vi "SMU_gate_2_constant.vi"() -> ()   [LabVIEW 2022 SP3]
uses:
  <vilib>/Analysis/1siggen.llb/Ramp Pattern by Delta.vi
  Agilent U2722/Public/Configure/Configure Channel (Current).vi
  Agilent U2722/Public/Configure/Configure Channel (Voltage).vi
  Agilent U2722/Public/Data/Read Output (Single).vi
  <vilib>/Utility/file.llb/Write Delimited Spreadsheet (DBL).vi
  Agilent U2722/Agilent U2722.lvlib
  <vilib>/Analysis/NI_AALBase.lvlib
panel:
  in  "Tab Control":enum32{"Device Setup"}(tab)
  out "V_out (V)":dbl
  out "I_measure_channel (A)":dbl
  out "Vdd (V)":dbl
  in  "Voltage Range 2":u16(ring) items=["2 Volts", "20 Volts"]
  in  "Current Range 2":u16(ring)=4 items=["1 uA", "10 uA", "100 uA", "1 mA", "10 mA", "120 mA"]
  in  "Current Limit  2":dbl=0.005 format="%#_2p"
  in  "Voltage Range":u16(ring) items=["2 Volts", "20 Volts"]
  in  "Starting Voltage (V)":dbl
  in  "Stopping Voltage (V)":dbl=1.0
  in  "Voltage Interval  (DV)":dbl format="%#_2g"
  in  "Current Range":u16(ring)=4 items=["1 uA", "10 uA", "100 uA", "1 mA", "10 mA", "120 mA"]
  in  "VISA resource name SMU 1":refnum<visa-resource-name>
  in  "Gate 1 Channel Config":u16(ring)=1 items=["Channel 1"=1, "Channel 2"=2, "Channel 3"=3]
  in  "PLC":i32
  in  "Current Limit":dbl=0.005 format="%#_2p"
  in  "Interval Time (s)":dbl=1.0 caption="Delay Time (s)"
  in  "Vdd Channel Config":u16(ring)=2 items=["Channel 1"=1, "Channel 2"=2, "Channel 3"=3]
  in  "output file path":path
  out "XY Graph":cluster{"Y":dbl[], "Y":dbl[]}[](graph)
  in  "VISA resource name SMU 2":refnum<visa-resource-name>
  in  "Voltage Range 3":u16(ring) items=["2 Volts", "20 Volts"]
  in  "Current Range 3":u16(ring)=4 items=["1 uA", "10 uA", "100 uA", "1 mA", "10 mA", "120 mA"]
  in  "Gate 2 Channel Config":u16(ring)=1 items=["Channel 1"=1, "Channel 2"=2, "Channel 3"=3]
  in  "PLC 2":i32
  in  "Current Limit  3":dbl=0.005 format="%#_2p"
  in  "Output Measure Channel Config":u16(ring)=2 items=["Channel 1"=1, "Channel 2"=2, "Channel 3"=3]
  in  "Vdd (V)":dbl
  in  "Gate 2 Voltage (V)":dbl
  out "Idd (A)":dbl
  # "Gate 1 Sweep Settings"
  # "Vdd Voltage Setting"
  # "Should be 0!"
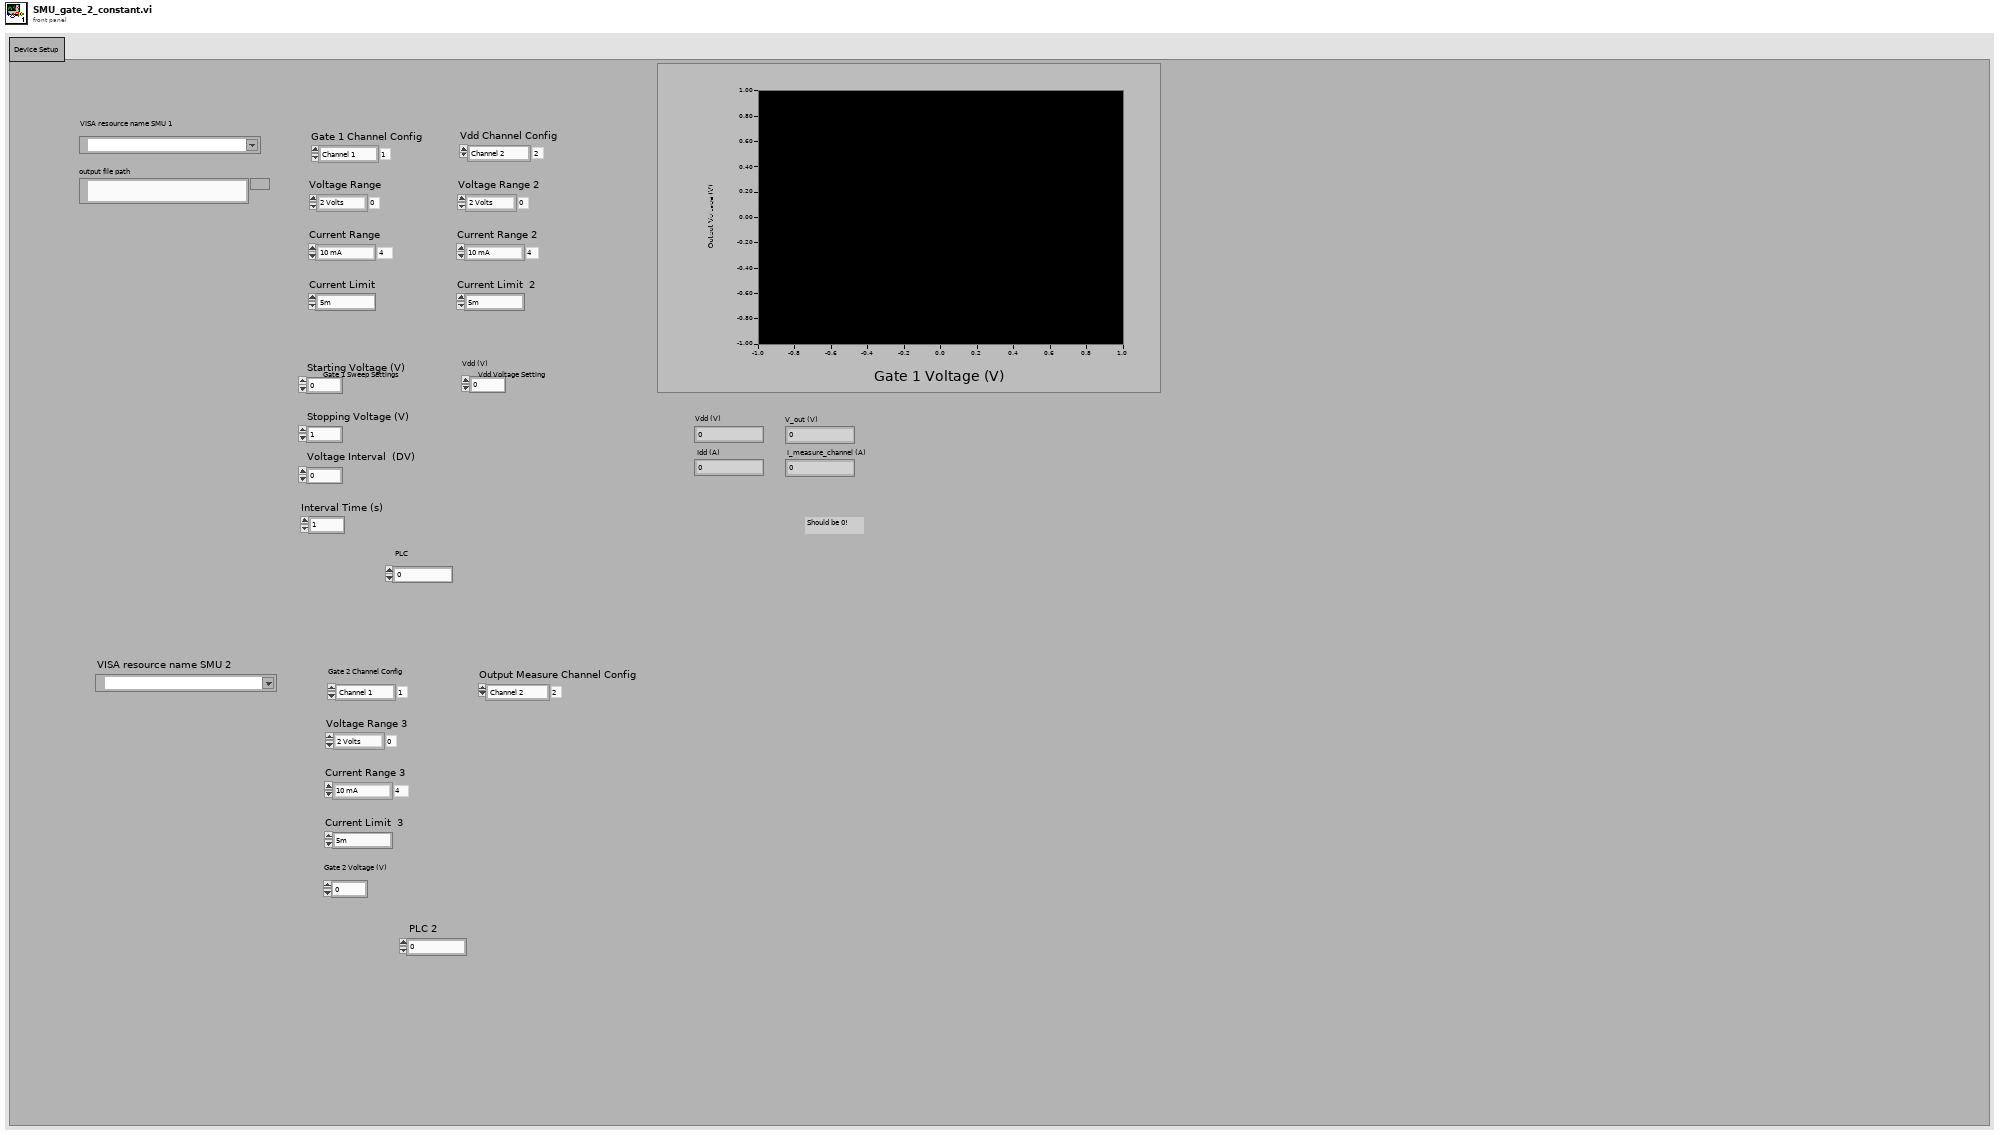
[diagram p1: front panel]
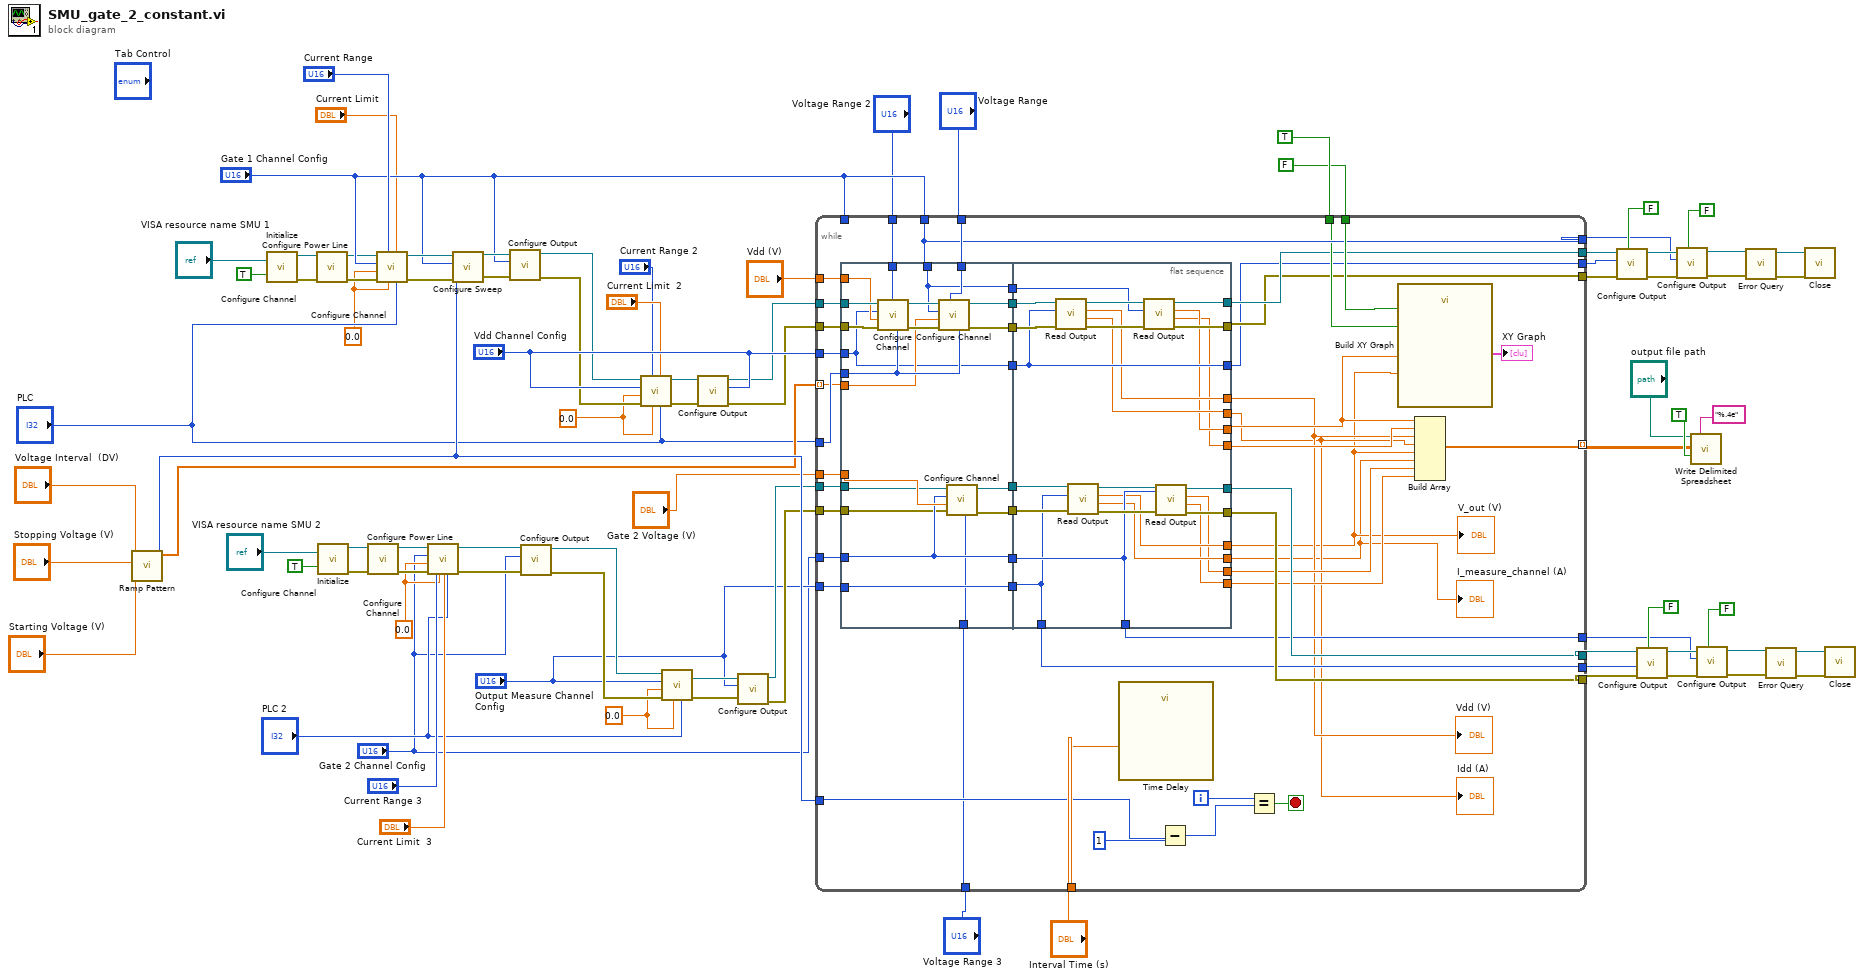
[diagram p0: block diagram]
diagram:
  w31 = 0.0
  w30 = 0.0
  w45 = 0.0
  w44 = 0.0
  n1 = call-poly <vilib>:"Ramp Pattern.vi"("start"="Starting Voltage (V)", "end"="Stopping Voltage (V)", "delta"="Voltage Interval  (DV)") -> ("samples"=w72:i32, "Ramp Pattern"=w64:dbl[])  [unwired: 6 in, 1 out]
  n2 = call "Initialize.vi"("ID Query (True)"=TRUE, "VISA resource name"="VISA resource name SMU 1") -> ("error out"=w82:errorcluster, "VISA resource name out"=w81:refnum<visa-resource-name>)  [unwired: 8 in]
  n3 = call "Configure Power Line.vi"("error in (no error)"=w82, "VISA resource name"=w81) -> ("error out"=w68:errorcluster, "VISA resource name out"=w61:refnum<visa-resource-name>)  [unwired: 8 in]
  n4 = call "Initialize.vi"("ID Query (True)"=TRUE, "VISA resource name"="VISA resource name SMU 2") -> ("error out"=w40:errorcluster, "VISA resource name out"=w39:refnum<visa-resource-name>)  [unwired: 8 in]
  n5 = call "Configure Power Line.vi"("error in (no error)"=w40, "VISA resource name"=w39) -> ("error out"=w38:errorcluster, "VISA resource name out"=w36:refnum<visa-resource-name>)  [unwired: 8 in]
  n6 = call-poly "Configure Channel.vi"("Power Line Cycles (0)"="PLC", "Current Limit (1.0 uA)"="Current Limit", "Triggered Level (1.0 mA)"=w44, "Current Range (0: 1 uA)"="Current Range", "error in (no error)"=w68, "Output Level (1.0 mA)"=w44, "Channel (1: Channel 1)"="Gate 1 Channel Config", "VISA resource name"=w61) -> ("error out"=w69:errorcluster, "VISA resource name out"=w70:refnum<visa-resource-name>)  [unwired: 2 in]
  n7 = call-poly "Configure Channel.vi"("Power Line Cycles (0)"="PLC 2", "Current Limit (1.0 uA)"="Current Limit  3", "Triggered Level (1.0 mA)"=w30, "Current Range (0: 1 uA)"="Current Range 3", "error in (no error)"=w38, "Output Level (1.0 mA)"=w30, "Channel (1: Channel 1)"="Gate 2 Channel Config", "VISA resource name"=w36) -> ("error out"=w20:errorcluster, "VISA resource name out"=w21:refnum<visa-resource-name>)  [unwired: 2 in]
  n8 = call "Configure Sweep.vi"("error in (no error)"=w69, "Sweep Points (1)"=w72, "Channel (1: Channel 1)"="Gate 1 Channel Config", "VISA resource name"=w70) -> ("error out"=w73:errorcluster, "VISA resource name out"=w74:refnum<visa-resource-name>)  [unwired: 6 in]
  n9 = call "Configure Output.vi"("error in (no error)"=w73, "Channel (1: Channel 1)"="Gate 1 Channel Config", "VISA resource name"=w74) -> ("error out"=w59:errorcluster, "VISA resource name out"=w60:refnum<visa-resource-name>)  [unwired: 7 in]
  n10 = call "Configure Output.vi"("error in (no error)"=w20, "Channel (1: Channel 1)"="Gate 2 Channel Config", "VISA resource name"=w21) -> ("error out"=w34:errorcluster, "VISA resource name out"=w35:refnum<visa-resource-name>)  [unwired: 7 in]
  n11 = call-poly "Configure Channel.vi"("Power Line Cycles (0)"="PLC", "Current Limit (1.0 uA)"="Current Limit  2", "Triggered Level (1.0 mA)"=w45, "Current Range (0: 1 uA)"="Current Range 2", "error in (no error)"=w59, "Output Level (1.0 mA)"=w45, "Channel (1: Channel 1)"="Vdd Channel Config", "VISA resource name"=w60) -> ("error out"=w25:errorcluster, "VISA resource name out"=w26:refnum<visa-resource-name>)  [unwired: 2 in]
  n12 = call-poly "Configure Channel.vi"("Power Line Cycles (0)"="PLC 2", "Triggered Level (1.0 mA)"=w31, "error in (no error)"=w34, "Output Level (1.0 mA)"=w31, "Channel (1: Channel 1)"="Output Measure Channel Config", "VISA resource name"=w35) -> ("error out"=w22:errorcluster, "VISA resource name out"=w23:refnum<visa-resource-name>)  [unwired: 4 in]
  n13 = call "Configure Output.vi"("error in (no error)"=w25, "Channel (1: Channel 1)"="Vdd Channel Config", "VISA resource name"=w26) -> ("error out"=w58:errorcluster, "VISA resource name out"=w57:refnum<visa-resource-name>)  [unwired: 7 in]
  n14 = call "Configure Output.vi"("error in (no error)"=w22, "Channel (1: Channel 1)"="Output Measure Channel Config", "VISA resource name"=w23) -> ("error out"=w18:errorcluster, "VISA resource name out"=w19:refnum<visa-resource-name>)  [unwired: 7 in]
  n15 = while {
    tunnel: w72 -> [w133]
    tunnel: "Interval Time (s)" -> [w132]
    tunnel: "PLC" -> [w117]
    tunnel: TRUE -> [w111]
    tunnel: FALSE -> [w127]
    tunnel: [w108] -> w66
    tunnel: [w107] -> w65
    tunnel: "Vdd Channel Config" -> [w122]
    tunnel: "Voltage Range" -> [w119]
    tunnel: "Vdd (V)" -> [w121]
    tunnel: [w128] -> w1 mode=indexing
    tunnel: w64 -> [w116] mode=indexing
    tunnel: "Gate 1 Channel Config" -> [_]
    tunnel: "Gate 1 Channel Config" -> [w118]
    tunnel: w57 -> [w124]
    tunnel: [w106] -> w51
    tunnel: [w118] -> w50
    tunnel: w58 -> [w123]
    tunnel: "Voltage Range 2" -> [w120]
    tunnel: w19 -> [w110]
    tunnel: w18 -> [w109]
    tunnel: [w105] -> w9
    tunnel: [w104] -> w8
    tunnel: "Output Measure Channel Config" -> [w103]
    tunnel: "Gate 2 Voltage (V)" -> [w102]
    tunnel: "Gate 2 Channel Config" -> [w100]
    tunnel: [w98] -> w5
    tunnel: [w97] -> w4
    tunnel: "Voltage Range 3" -> [w96]
    i -> [w130]
    stop <- w131 stop-if-true
    n16 = flat-sequence {
      tunnel: [w155] -> w126
      tunnel: [w153] -> w125
      tunnel: w124 -> [w152]
      tunnel: w123 -> [w151]
      tunnel: w122 -> [w145]
      tunnel: w121 -> [w150]
      tunnel: w120 -> [w149]
      tunnel: w119 -> [w148]
      tunnel: w118 -> [w144]
      tunnel: w117 -> [w147]
      tunnel: w116 -> [w146]
      tunnel: [w145] -> w115
      tunnel: [w144] -> w114
      tunnel: [w143] -> w113
      tunnel: [w142] -> w112
      tunnel: w110 -> [w137]
      tunnel: w109 -> [w136]
      tunnel: w103 -> [w140]
      tunnel: w102 -> [w141]
      tunnel: [w140] -> w101
      tunnel: w100 -> [w139]
      tunnel: [w139] -> w99
      tunnel: w96 -> [w138]
      tunnel: w126 -> [w180]
      tunnel: [w178] -> w108
      tunnel: w125 -> [w177]
      tunnel: [w175] -> w107
      tunnel: w115 -> [w167]
      tunnel: w114 -> [w174]
      tunnel: w113 -> [w173]
      tunnel: w112 -> [w171]
      tunnel: [w169] -> w105
      tunnel: [w168] -> w104
      tunnel: [w167] -> w106
      tunnel: w101 -> [w165]
      tunnel: w99 -> [w166]
      tunnel: [w166] -> w98
      tunnel: [w165] -> w97
      tunnel: [w164] -> w91
      tunnel: [w163] -> w90
      tunnel: [w162] -> w95
      tunnel: [w161] -> w94
      tunnel: [w160] -> w89
      tunnel: [w159] -> w88
      tunnel: [w158] -> w93
      tunnel: [w157] -> w92
      frame #0 {
        n17 = call-poly "Configure Channel.vi"("Power Line Cycles (0)"=w147, "Voltage Range (0: 2 Volts)"=w149, "error in (no error)"=w151, "Output Level (1.0 V)"=w150, "Channel (1: Channel 1)"=w145, "VISA resource name"=w152) -> ("error out"=w154:errorcluster, "VISA resource name out"=w156:refnum<visa-resource-name>)  [unwired: 4 in]
        n18 = call-poly "Configure Channel.vi"("Power Line Cycles (0)"=w147, "Voltage Range (0: 2 Volts)"=w148, "error in (no error)"=w154, "Output Level (1.0 V)"=w146, "Channel (1: Channel 1)"=w144, "VISA resource name"=w156) -> ("error out"=w153:errorcluster, "VISA resource name out"=w155:refnum<visa-resource-name>)  [unwired: 4 in]
        n19 = call-poly "Configure Channel.vi"("Voltage Range (0: 2 Volts)"=w138, "error in (no error)"=w136, "Output Level (1.0 V)"=w141, "Channel (1: Channel 1)"=w139, "VISA resource name"=w137) -> ("error out"=w142:errorcluster, "VISA resource name out"=w143:refnum<visa-resource-name>)  [unwired: 5 in]
      }
      frame #1 {
        n20 = call-poly "Read Output.vi"("error in (no error)"=w177, "Channel (1: Channel 1)"=w167, "VISA resource name"=w180) -> ("error out"=w176:errorcluster, "Actual Current Level (A)"=w163:dbl, "Actual Voltage Level (V)"=w164:dbl, "VISA resource name out"=w179:refnum<visa-resource-name>)  [unwired: 5 in]
        n21 = call-poly "Read Output.vi"("error in (no error)"=w171, "Channel (1: Channel 1)"=w165, "VISA resource name"=w173) -> ("error out"=w170:errorcluster, "Actual Current Level (A)"=w159:dbl, "Actual Voltage Level (V)"=w160:dbl, "VISA resource name out"=w172:refnum<visa-resource-name>)  [unwired: 5 in]
        n22 = call-poly "Read Output.vi"("error in (no error)"=w176, "Channel (1: Channel 1)"=w174, "VISA resource name"=w179) -> ("error out"=w175:errorcluster, "Actual Current Level (A)"=w161:dbl, "Actual Voltage Level (V)"=w162:dbl, "VISA resource name out"=w178:refnum<visa-resource-name>)  [unwired: 5 in]
        n23 = call-poly "Read Output.vi"("error in (no error)"=w170, "Channel (1: Channel 1)"=w166, "VISA resource name"=w172) -> ("error out"=w168:errorcluster, "Actual Current Level (A)"=w157:dbl, "Actual Voltage Level (V)"=w158:dbl, "VISA resource name out"=w169:refnum<visa-resource-name>)  [unwired: 5 in]
      }
    }
    n24 = call "Time Delay"("Delay Time (s)"=w132) -> ()  [unwired: 10 in, 1 out]
    n25 = Subtract(x=w133, y=1 ("x")) -> (x-y=w134:i32)
    n26 = Equal?(x=w130, y=w134) -> (x = y?=w131:bool)
    n27 = call "Build XY Graph"("Enable"=w111, "Reset"=w127, "Y Input"=w89, "X Input"=w95) -> ("XY Graph"=→"XY Graph":cluster{"X":dbl[], "Y":dbl[]}[])  [unwired: 6 in, 1 out]
    n28 = Build Array(w95, w94, w91, w90, w89, w88, w93, w92) -> (w128:dbl[])
    "Vdd (V)" <- w91
    "Idd (A)" <- w90
    "I_measure_channel (A)" <- w88
    "V_out (V)" <- w89
  }
  n29 = call "Configure Output.vi"("Enable Output (T: Enable)"=FALSE, "error in (no error)"=w65, "Channel (1: Channel 1)"=w51, "VISA resource name"=w66) -> ("error out"=w54:errorcluster, "VISA resource name out"=w56:refnum<visa-resource-name>)  [unwired: 6 in]
  n30 = call "Configure Output.vi"("Enable Output (T: Enable)"=FALSE, "error in (no error)"=w8, "Channel (1: Channel 1)"=w4, "VISA resource name"=w9) -> ("error out"=w12:errorcluster, "VISA resource name out"=w14:refnum<visa-resource-name>)  [unwired: 6 in]
  n31 = call "Configure Output.vi"("Enable Output (T: Enable)"=FALSE, "error in (no error)"=w54, "Channel (1: Channel 1)"=w50, "VISA resource name"=w56) -> ("error out"=w53:errorcluster, "VISA resource name out"=w55:refnum<visa-resource-name>)  [unwired: 6 in]
  n32 = call-poly <vilib>:"Write Delimited Spreadsheet.vi"("file path (dialog if empty)"="output file path", "format (%.3f)"="%.4e", "2D data"=w1, "append to file? (new file:F)"=TRUE) -> ()  [unwired: 10 in, 2 out]
  n33 = call "Configure Output.vi"("Enable Output (T: Enable)"=FALSE, "error in (no error)"=w12, "Channel (1: Channel 1)"=w5, "VISA resource name"=w14) -> ("error out"=w11:errorcluster, "VISA resource name out"=w13:refnum<visa-resource-name>)  [unwired: 6 in]
  n34 = call "Error Query.vi"("error in (no error)"=w53, "VISA resource name"=w55) -> ("error out"=w76:errorcluster, "VISA resource name out"=w75:refnum<visa-resource-name>)  [unwired: 6 in, 2 out]
  n35 = call "Error Query.vi"("error in (no error)"=w11, "VISA resource name"=w13) -> ("error out"=w16:errorcluster, "VISA resource name out"=w15:refnum<visa-resource-name>)  [unwired: 6 in, 2 out]
  n36 = call "Close.vi"("error in (no error)"=w76, "VISA resource name"=w75) -> ()  [unwired: 9 in, 1 out]
  n37 = call "Close.vi"("error in (no error)"=w16, "VISA resource name"=w15) -> ()  [unwired: 9 in, 1 out]
